vi "Send Perform Action.vi"(5 "DataSocket IP":string="dstp://192.168.0.1/fan1", 7 "Message Priority (Normal)":T1=enum."Normal", 8 "error in":errorcluster, 9 "Input":variant, 10 "Point Ident":string, 11 "Message Enqueuer":refnum<class "Message Enqueuer.lvclass">) -> (0 "error out":errorcluster, 1 "Output":variant, 2 "timed out?":bool, 3 "Message Enqueuer out":refnum<class "Message Enqueuer.lvclass">)   [LabVIEW 2023, in "IMSS Target Actor.lvlib" / "Perform Action Msg.lvclass"]
doc: "This VI sends the message to an actor."
uses:
  Perform Action Msg.lvclass
  <vilib>/ActorFramework/Message Enqueuer/Message Enqueuer.lvclass
  <vilib>/ActorFramework/Message Enqueuer/Message Priority.ctl
  Perform Action Msg.lvclass/Perform Action Msg.ctl
  DS-Reply-Msg/DS Reply Msg/DS Reply Msg.lvclass
  D:/git/DS-Reply-Msg/DS Reply Msg/DS Reply Msg.lvclass
  C:/Program Files/National Instruments/LabVIEW 2023/vi.lib/ActorFramework/Message/Message.lvclass
  D:/git/HAL/HAL GOOP4/MSS Target/IMSS Target Actor Messages/Perform Action Msg/Perform Action Msg.lvclass
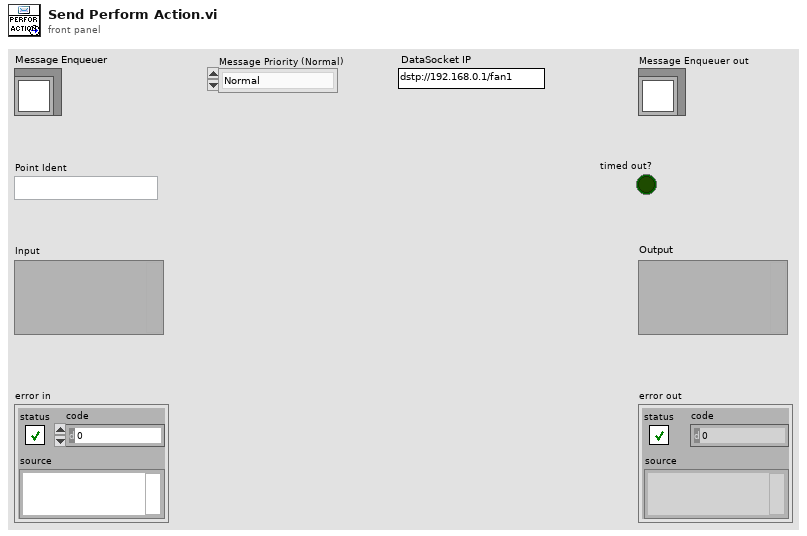
[diagram p1: front panel]
types:
  T1 = typedef "Actor Framework.lvlib/Message Enqueuer.lvclass/Message Priority.ctl" = enum16{"Low", "Normal", "High"}
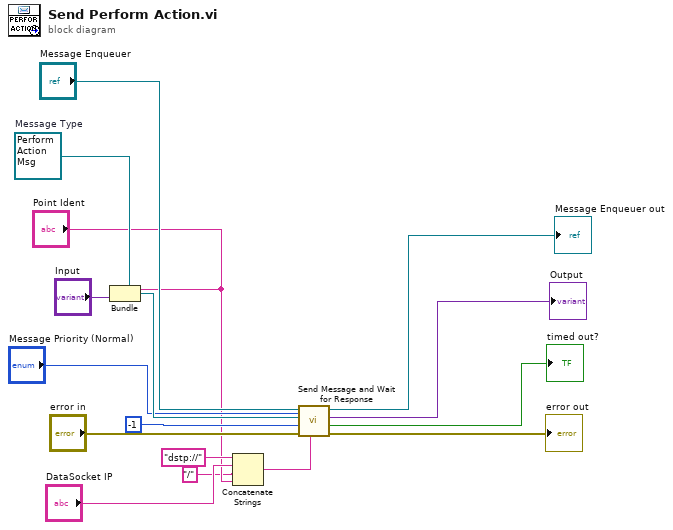
[diagram p0: block diagram]
diagram:
  w13 = refnum<class "Perform Action Msg.lvclass"> refnum  # Message Type
  n1 = Bundle(cluster=w13, "Point Ident", "Input") -> (w12:refnum<class "Perform Action Msg.lvclass">)
  n2 = Concatenate Strings("dstp://" ("string"), "DataSocket IP", "/" ("string"), "Point Ident") -> (w3:string)
  n3 = call "Send Message and Wait for Response.vi"("DataSocket Location"=w3, "Message Priority (Normal)"="Message Priority (Normal)", "error in"="error in", "timeout in ms (-1)"=-1, "Original Message"=w12, "Message Enqueuer in"="Message Enqueuer") -> ("error out"=→"error out":errorcluster, "timed out?"=→"timed out?":bool, "Reply"=→"Output":variant, "Message Enqueuer out"=→"Message Enqueuer out":refnum<class "Message Enqueuer.lvclass">)  [unwired: 2 in]
